vi "set_galvo_voltages.vi"(4 "deltaVy0(V)":dbl, 6 "Vy0(V)":dbl, 8 "error in (no error)":errorcluster, 9 "deltaVz(V)":dbl, 10 "Vz0(V)":dbl, 11 "TrajectoryAK101022Resonance in":refnum<class "TrajectoryAK101022Resonance.lvclass">) -> (0 "error out":errorcluster, 3 "TrajectoryAK101022Resonance out":refnum<class "TrajectoryAK101022Resonance.lvclass">)   [LabVIEW 2010, in "TrajectoryAK101022Resonance.lvclass"]
uses:
  TrajectoryAK101022Resonance.lvclass
  TrajectoryAK101022Resonance.lvclass/TrajectoryAK101022Resonance.ctl
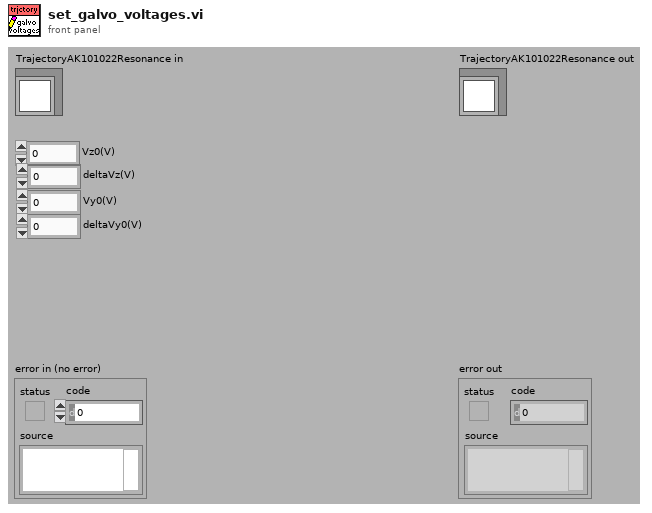
[diagram p1: front panel]
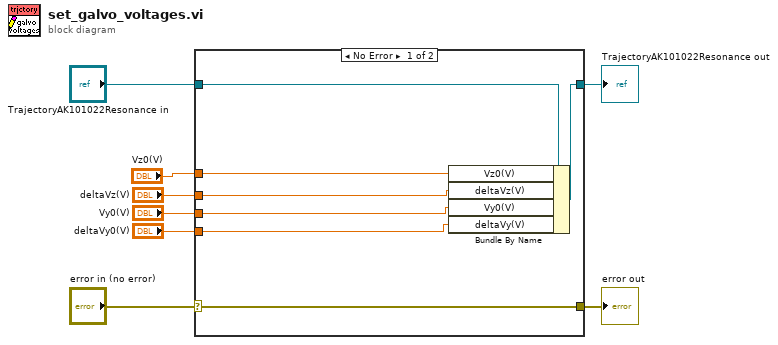
[diagram p0: block diagram]
diagram:
  n1 = case shown="No Error" "error in (no error)" {
    selector: "error in (no error)" -> [w15 w16]
    tunnel: [w15 w16] -> w7
    tunnel: [w13 w17] -> w5
    tunnel: "TrajectoryAK101022Resonance in" -> [w14 w17]
    tunnel: "Vz0(V)" -> [w12 _]
    tunnel: "deltaVz(V)" -> [w11 _]
    tunnel: "Vy0(V)" -> [w10 _]
    tunnel: "deltaVy0(V)" -> [w9 _]
    frame No Error {
      n2 = Bundle By Name(cluster=w14, "Vz0(V)"=w12, "deltaVz(V)"=w11, "Vy0(V)"=w10, "deltaVy(V)"=w9) -> (w13:refnum<class "TrajectoryAK101022Resonance.lvclass">)
    }
    frame Error {
    }
  }
  "error out" <- w7
  "TrajectoryAK101022Resonance out" <- w5
